vi "loadBfieldFromFile.vi"(11 "index":i32) -> (0 "spec cluster 2":cluster{dbl[], dbl[]}[](graph), 1 "change from file":dbl, 2 "spec cluster":cluster{dbl[], dbl[]}(graph), 3 "B [T]":dbl)   [LabVIEW 2011]
uses:
  NI_AALPro.lvlib
panel:
  out "path 2":path
  out "all rows 4":string[][](array[string])
  out "deleted portion":string[](array[string])
  out "result":dbl format="%0.4f"
  out "path":path
  out "all rows 3":string[][](array[string])
  out "all rows 2":string[][](array[string])
  out "subarray":string[](array[string])
  out "all rows":string[][](array[string])
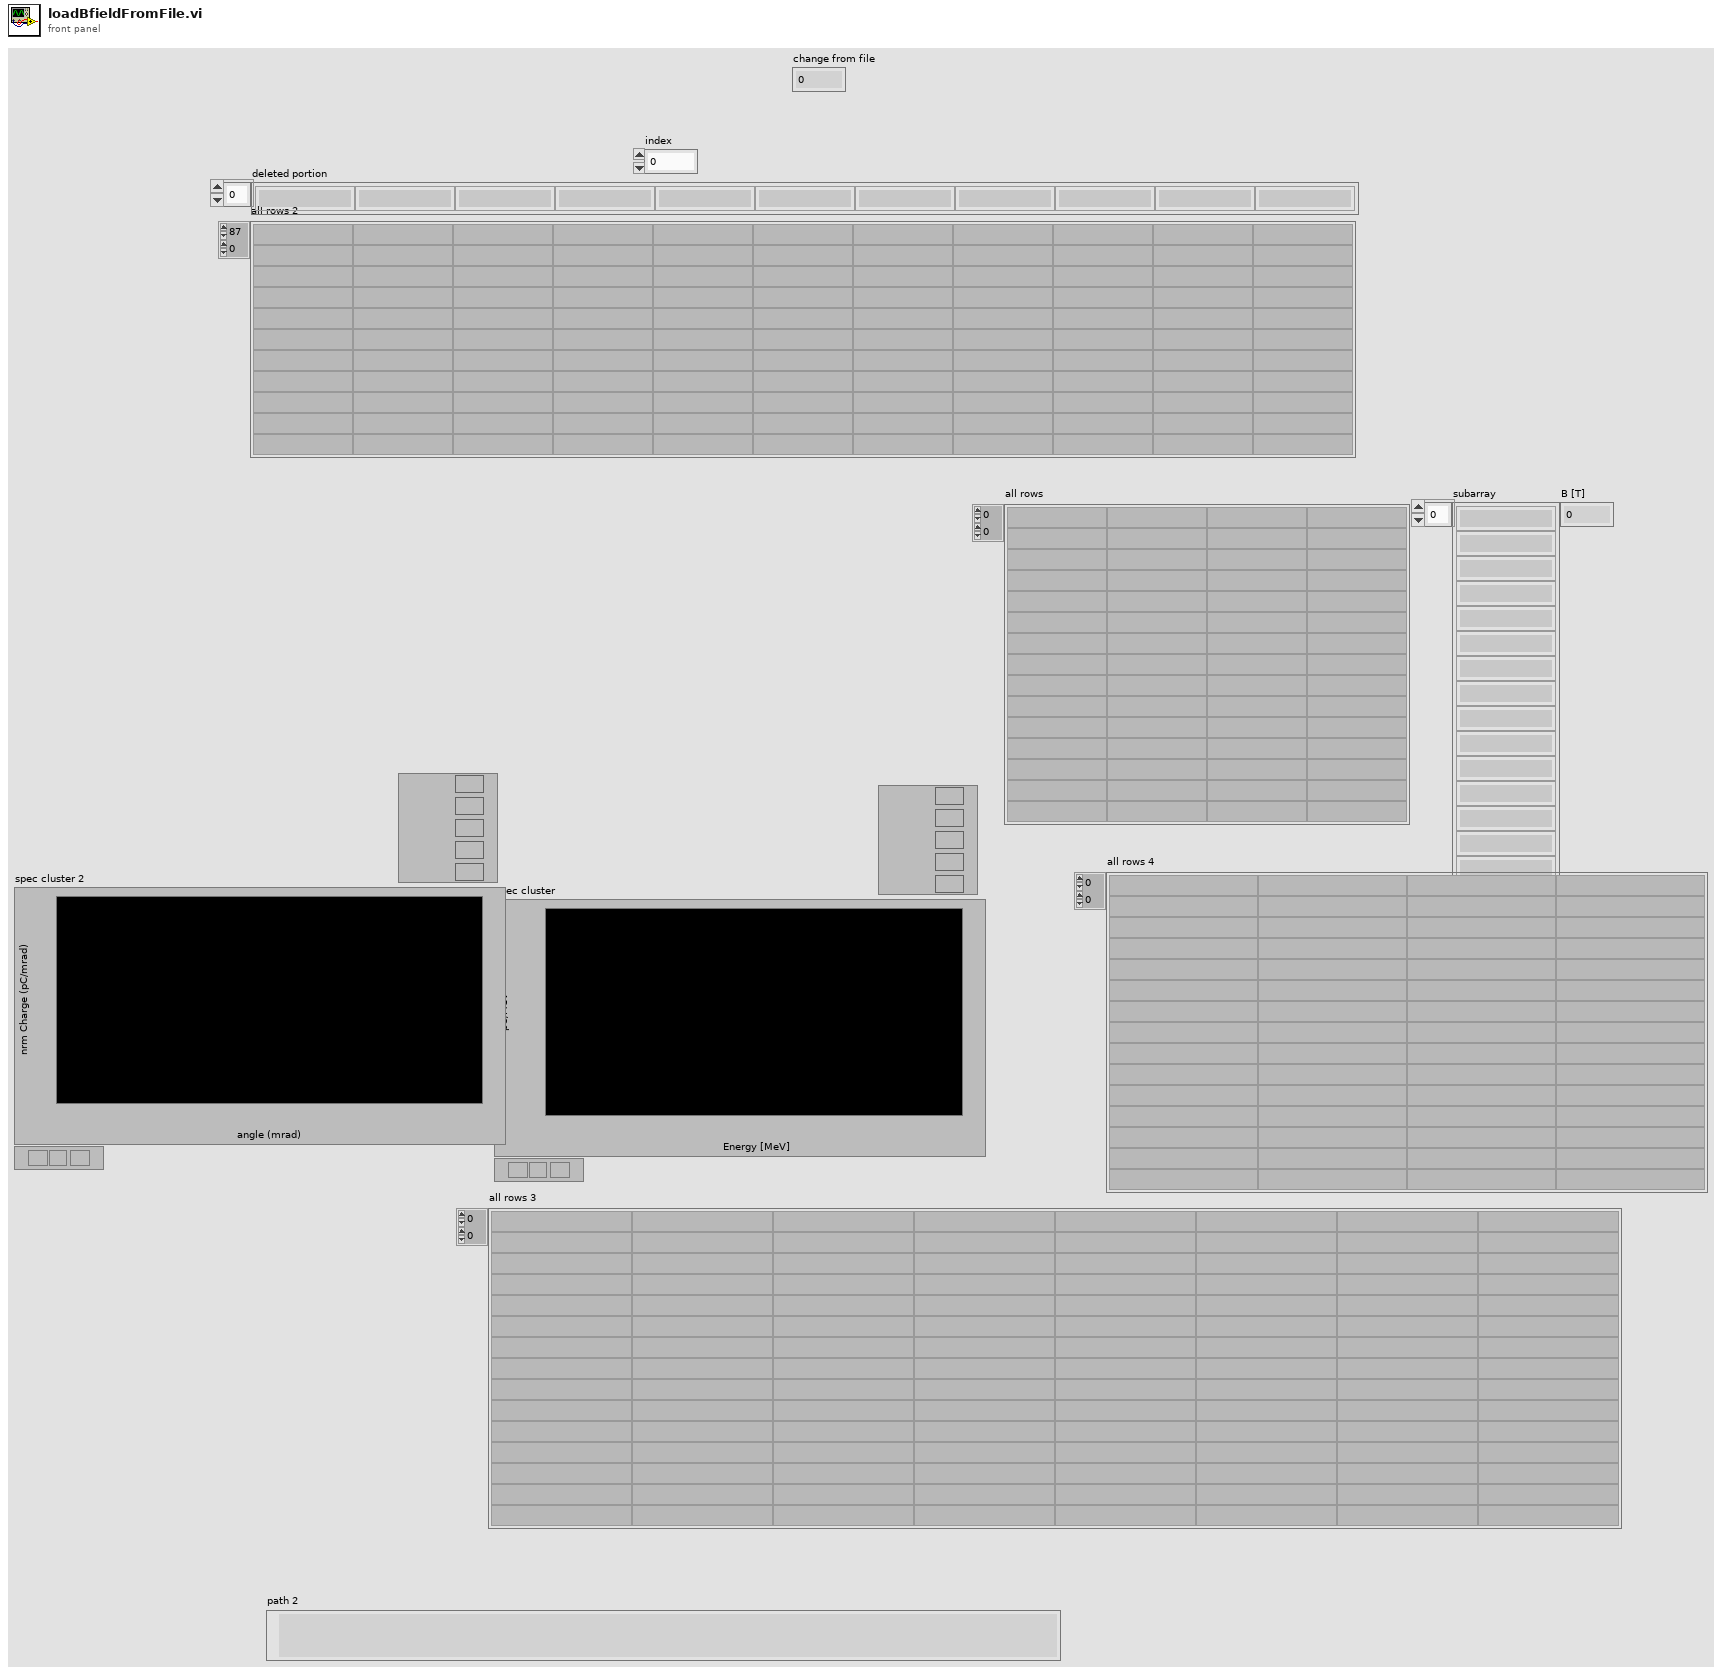
[diagram p1: front panel]
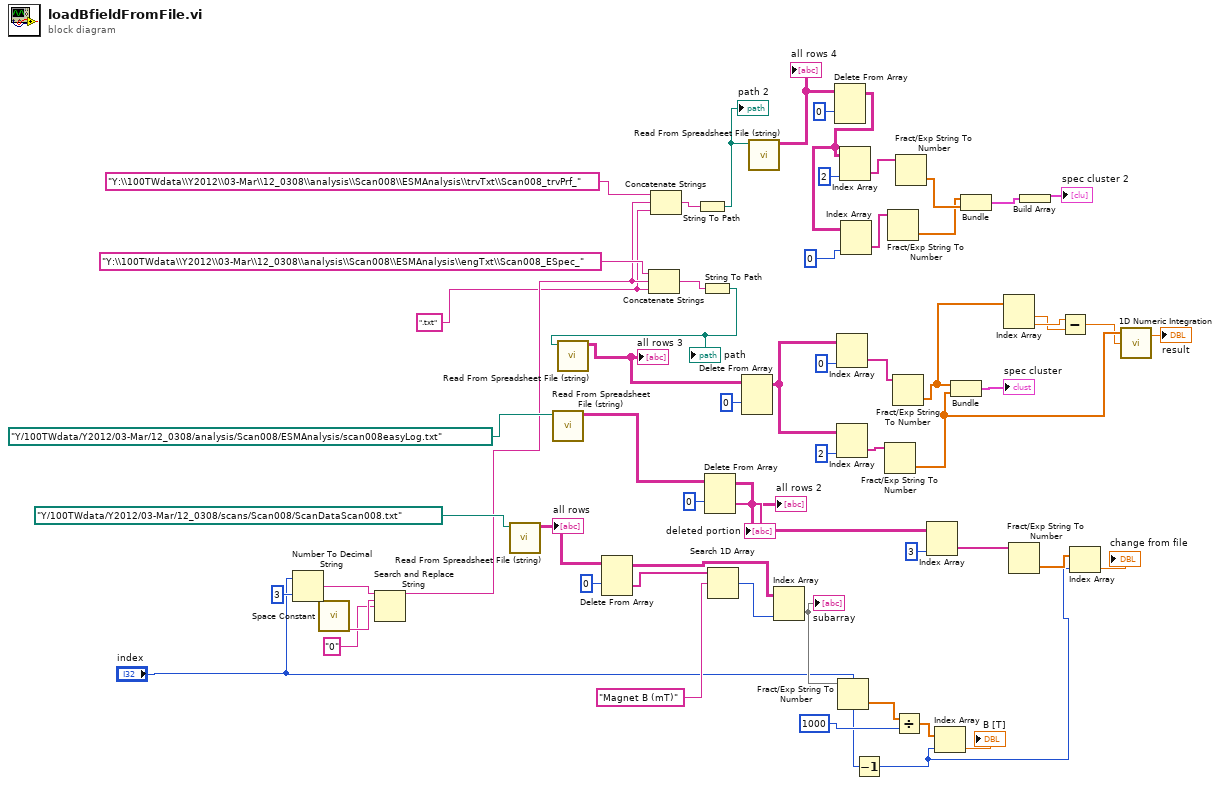
[diagram p0: block diagram]
diagram:
  w9 = ".txt"
  n1 = Number To Decimal String(number="index", width (-)=i16 3) -> (decimal integer string=w39:string)
  n2 = call "Space Constant.vi"() -> ("String"=w38:string)
  n3 = Search and Replace String(input string=w39, search string=w38, replace string="0") -> (result string=w10:string)  [unwired: 5 in, 3 out]
  n4 = call "Read From Spreadsheet File (string).vi"("file path (dialog if empty)"=path "Y:/100TWdata/Y2012/03-Mar/12_0308/scans/Scan008/ScanDataScan008.txt" ("path")) -> ("all rows"=w59:string[][])  [unwired: 6 in, 4 out]
  "all rows" <- w59
  n5 = call "Read From Spreadsheet File (string).vi"("file path (dialog if empty)"=path "Y:/100TWdata/Y2012/03-Mar/12_0308/analysis/Scan008/ESMAnalysis/scan008easyLog.txt" ("path")) -> ("all rows"=w28:string[][])  [unwired: 6 in, 4 out]
  n6 = Delete From Array(array=w59, index (row)=0) -> (deleted portion=w57:string[], array with subset deleted=w55:string[][])  [unwired: 2 in]
  n7 = Concatenate Strings("Y:\\100TWdata\\Y2012\\03-Mar\\12_0308\\analysis\\Scan008\\ESMAnalysis\\engTxt\\Scan008_ESpec_", w10, w9) -> (w35:string)
  n8 = Concatenate Strings("Y:\\100TWdata\\Y2012\\03-Mar\\12_0308\\analysis\\Scan008\\ESMAnalysis\\trvTxt\\Scan008_trvPrf_", w10, w9) -> (w8:string)
  n9 = String To Path(string=w8) -> (path=w7:path)
  "path 2" <- w7
  n10 = String To Path(string=w35) -> (path=w34:path)
  "path" <- w34
  n11 = call "Read From Spreadsheet File (string).vi"("file path (dialog if empty)"=w34) -> ("all rows"=w46:string[][])  [unwired: 6 in, 4 out]
  "all rows 3" <- w46
  n12 = Delete From Array(array=w28, index (row)=0) -> (deleted portion=→"deleted portion":string[], array with subset deleted=w24:string[][])  [unwired: 2 in]
  "all rows 2" <- w24
  n13 = Search 1D Array(1D array=w57, element="Magnet B (mT)") -> (index of element=w54:i32)  [unwired: 1 in]
  n14 = Delete From Array(array=w46, index (row)=0) -> (array with subset deleted=w16:string[][])  [unwired: 2 in, 1 out]
  n15 = call "Read From Spreadsheet File (string).vi"("file path (dialog if empty)"=w7) -> ("all rows"=w5:string[][])  [unwired: 6 in, 4 out]
  "all rows 4" <- w5
  n16 = Index Array(array=w55, index (col)=w54) -> (element=w53:string[])  [unwired: 1 in]
  "subarray" <- w53
  n17 = Delete From Array(array=w5, index (row)=0) -> (array with subset deleted=w3:string[][])  [unwired: 2 in, 1 out]
  n18 = Index Array(array=w16, index (col)=0 ("disabled index (col)")) -> (element=w43:string[])  [unwired: 1 in]
  n19 = Index Array(array=w16, index (col)=2 ("disabled index (col)")) -> (element=w42:string[])  [unwired: 1 in]
  n20 = Fract/Exp String To Number(string=w53) -> (number=w52:dbl[])  [unwired: 3 in, 1 out]
  n21 = Index Array(array=w3, index (col)=2 ("disabled index (col)")) -> (element=w15:string[])  [unwired: 1 in]
  n22 = Index Array(array=w3, index (col)=0 ("index (row)")) -> (element=w1:string[])  [unwired: 1 in]
  n23 = Decrement(x="index") -> (x-1=w19:i32)
  n24 = Fract/Exp String To Number(string=w42) -> (number=w31:dbl[])  [unwired: 3 in, 1 out]
  n25 = Fract/Exp String To Number(string=w1) -> (number=w4:dbl[])  [unwired: 3 in, 1 out]
  n26 = Fract/Exp String To Number(string=w43) -> (number=w18:dbl[])  [unwired: 3 in, 1 out]
  n27 = Divide(x=w52, y=1000) -> (x/y=w50:dbl[])
  n28 = Fract/Exp String To Number(string=w15) -> (number=w14:dbl[])  [unwired: 3 in, 1 out]
  n29 = Index Array(array=w24, index (col)=3 ("disabled index (col)")) -> (element=w23:string[])  [unwired: 1 in]
  n30 = Index Array(array=w50, index=w19) -> (element=→"B [T]":dbl)
  n31 = Bundle(w18, w31) -> (→"spec cluster":cluster{dbl[], dbl[]})  [unwired: 1 in]
  n32 = Bundle(w4, w14) -> (w13:cluster{dbl[], dbl[]})  [unwired: 1 in]
  n33 = Index Array(array=w18) -> (element #1=w32:dbl, element #2=w33:dbl)  [unwired: 2 in]
  n34 = Fract/Exp String To Number(string=w23) -> (number=w22:dbl[])  [unwired: 3 in, 1 out]
  n35 = Build Array(w13) -> (→"spec cluster 2":cluster{dbl[], dbl[]}[])
  n36 = Subtract(x=w33, y=w32) -> (x-y=w30:dbl)
  n37 = Index Array(array=w22, index=w19) -> (element=→"change from file":dbl)
  n38 = call "1D Numeric Integration.vi"("dt"=w30, "Input Array"=w31) -> ("result"=→"result":dbl)  [unwired: 1 in, 1 out]
